vi "main.vi"() -> ()   [LabVIEW 2013]
panel:
  out "2Dピクチャ":picture
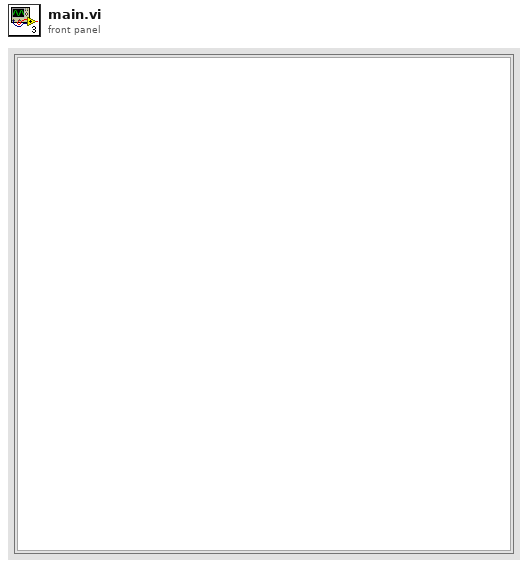
[diagram p1: front panel]
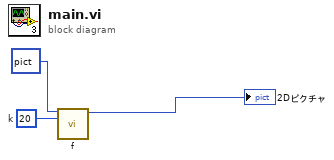
[diagram p0: block diagram]
diagram:
  w3 = 20  # k
  n1 = call "f.vi"("2Dピクチャ"=picture data[5B], "k"=w3) -> ("2Dピクチャ"=→"2Dピクチャ":picture)  [unwired: 12 in, 1 out]
